vi "MDPtr Pack WaveformArr.vi"(7 "Copies Count(1)":i32=1, 9 "String Attribute":string, 10 "error in (no error)":errorcluster, 11 "waveforms":waveform(dbl)[](array[waveform])) -> (2 "error out":errorcluster, 3 "HexStrPtr":T1)   [LabVIEW 2017]
uses:
  MDPtr TypeDef/MDPtr.ctl
  MDPtr TypeDef/MDPtr DataFrame-WaveformArr.ctl
  MDPtr TypeDef/MDPtr DataFrame-Common.ctl
  MDPtr TypeDef/MDPtr SupportedDataTypeDef.ctl
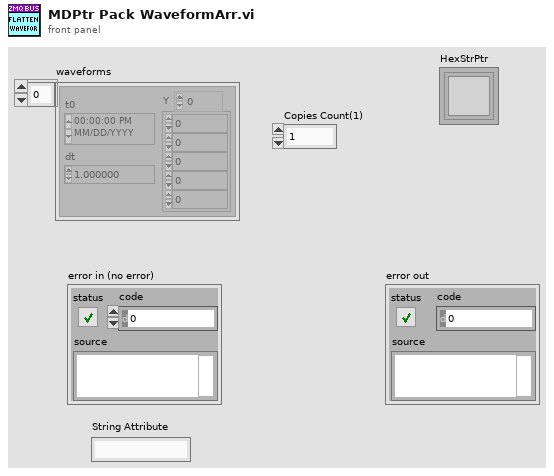
[diagram p1: front panel]
types:
  T1 = typedef "MDPtr.ctl" = refnum<k1>
  T2 = typedef "MDPtr SupportedDataTypeDef.ctl" = enum16{"<Invalid>", "<User 0>", "<User 1>", "<User 2>", "<User 3>", "<User 4>", "Memory", "Waveform", "Waveform Arr", "Double Arr", "String Arr"}
  T3 = typedef "MDPtr DataFrame-WaveformArr.ctl" = cluster{"Common":T4, "DVR":refnum<data-value>}
  T4 = typedef "MDPtr DataFrame-Common.ctl" = cluster{"Data Type":T2, "Copy Count":i32, "String Attribute":string}
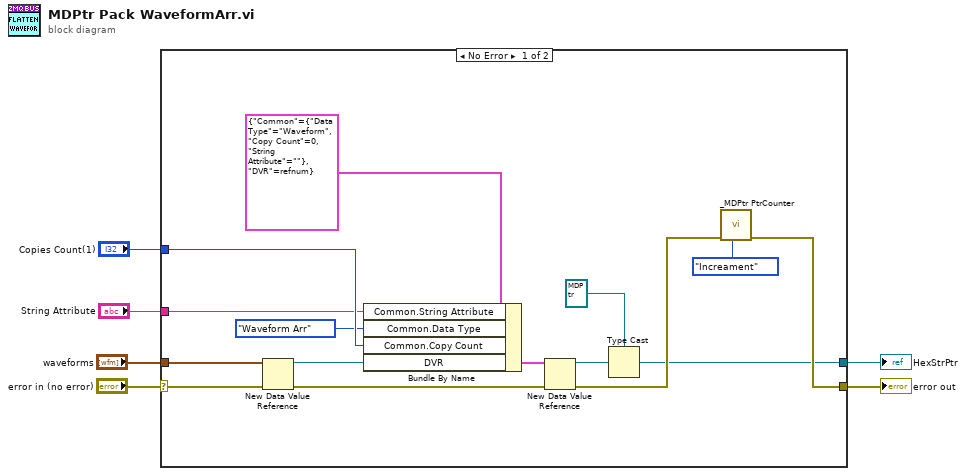
[diagram p0: block diagram]
diagram:
  n1 = case shown="No Error" "error in (no error)" {
    selector: "error in (no error)" -> [w19 w22]
    tunnel: [w15 w22] -> w5
    tunnel: "waveforms" -> [w13 _]
    tunnel: [w9 _] -> w3
    tunnel: "Copies Count(1)" -> [w11 _]
    tunnel: "String Attribute" -> [w7 _]
    frame No Error {
      n2 = New Data Value Reference(data value=w13, error in=w19) -> (data value reference=w12:refnum<data-value>, error out=w18:errorcluster)
      n3 = Bundle By Name(cluster=T3 {"Common"={"Data Type"=enum."Waveform", "Copy Count"=0, "String Attribute"=""}, "DVR"=refnum} ("output cluster"), "Common.String Attribute"=w7, "Common.Data Type"=MDPtr_SupportedDataTypeDef."Waveform Arr" ("Data Type"), "Common.Copy Count"=w11, "DVR"=w12) -> (w20:T3)
      n4 = New Data Value Reference(data value=w20, error in=w18) -> (data value reference=w14:refnum<data-value>, error out=w16:errorcluster)
      n5 = Type Cast(type=T1 refnum ("MDPtr"), x=w14) -> (*(type *) &x=w9:T1)
      n6 = call "_MDPtr PtrCounter.vi"("Oper(Get)"=enum16{"GET", "Increament", "decreament"}."Increament", "error in (no error)"=w16) -> ("error out"=w15:errorcluster)  [unwired: 8 in, 1 out]
    }
    frame Error {
    }
  }
  "HexStrPtr" <- w3
  "error out" <- w5
